vi "Configure Initiate Continuous.vi"(8 "error in (no error)":errorcluster, 10 "Continuous Initiate (F:Disable)":bool, 11 "VISA resource name":refnum<visa-resource-name>) -> (0 "error out":errorcluster, 3 "VISA resource name out":refnum<visa-resource-name>)   [LabVIEW 2019, in "Agilent E4980.lvlib"]
doc: "Enables or disables the automatic trigger, which changes the trigger state from \"Idle\" to \"Wait for Trigger\"."
uses:
  Agilent E4980.lvlib
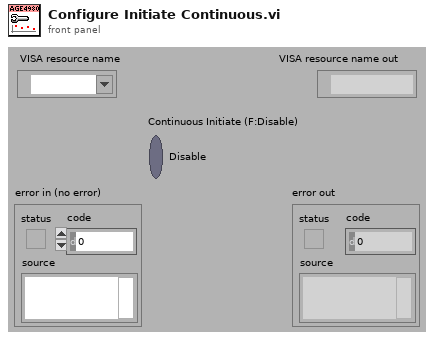
[diagram p1: front panel]
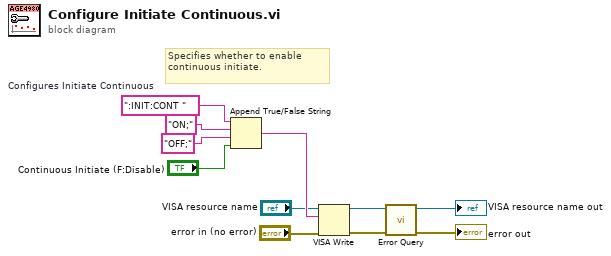
[diagram p0: block diagram]
diagram:
  w11 = ":INIT:CONT "  # Configures Initiate Continuous
  # "Specifies whether to enable\ncontinuous initiate."
  n1 = Append True/False String(1:"Continuous Initiate (F:Disable)", 2:"OFF;" ("false string"), 3:"ON;" ("true string"), 4:w11) -> (0:w6:string)
  n2 = VISA Write(VISA resource name="VISA resource name", write buffer=w6, error in (no error)="error in (no error)") -> (VISA resource name out=w5:refnum<visa-resource-name>, error out=w4:errorcluster)  [unwired: 1 out]
  n3 = call "Error Query.vi"("error in (no error)"=w4, "VISA resource name"=w5) -> ("error out"=→"error out":errorcluster, "VISA resource name out"=→"VISA resource name out":refnum<visa-resource-name>)  [unwired: 6 in, 2 out]
